vi "calibrationSpectrometer_logEvent_InternalCommand.vi"(8 "error in (no error)":errorcluster, 11 "logevent_InternalCommand_Ctl":T1) -> (0 "error out":errorcluster, 2 "function return":i32, 3 "logevent_InternalCommand_Ctl out":T1)   [LabVIEW 2016, in "SALLV_calibrationSpectrometer.lvlib"]
doc: "int calibrationSpectrometer_shm_logEvent_InternalCommandLV(calibrationSpectrometer_logevent_InternalCommandLV *logevent_InternalCommand_Ctl );"
uses:
  SALLV_calibrationSpectrometer.lvlib
  DataTypes/logevent_InternalCommand.ctl
  SALLV_calibrationSpectrometer.so
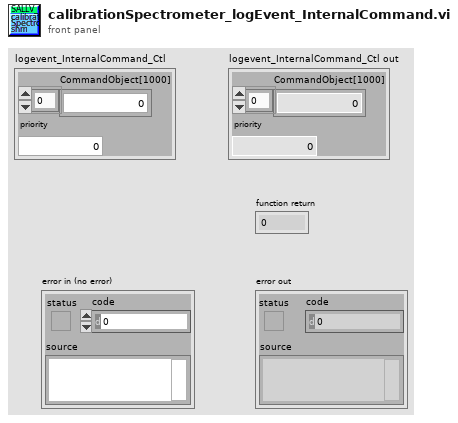
[diagram p1: front panel]
types:
  T1 = typedef "SALLV_calibrationSpectrometer.lvlib/logevent_InternalCommand.ctl" = cluster{"CommandObject[1000]":u8[], "priority":i32}
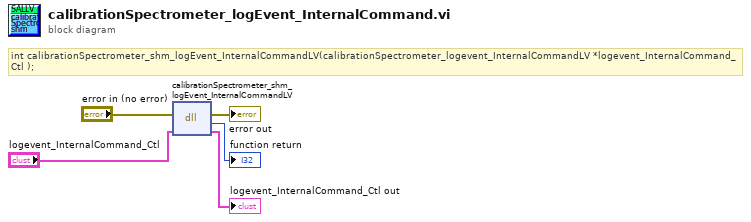
[diagram p0: block diagram]
diagram:
  # "int calibrationSpectrometer_shm_logEvent_InternalCommandLV(calibrationSpectrometer_logevent_InternalCommandLV *logevent_InternalCommand_Ctl );"
  n1 = dll-call lib="home/harini/TCS/sallv_sedspectrometer/SALLV_calibrationSpectrometer.*" fn="calibrationSpectrometer_shm_logEvent_InternalCommandLV"(error in="error in (no error)", "logevent_InternalCommand_Ctl"="logevent_InternalCommand_Ctl") -> (error out=→"error out":errorcluster, →"function return":i32, "logevent_InternalCommand_Ctl"=→"logevent_InternalCommand_Ctl out":T1)  [unwired: 2 in, 1 out]
